vi "PostBuild.vi"(5 "Files Generated\nby Build":path[](array[path]), 6 "Top Level/Always Included VIs":path[](array[path]), 7 "Destination Path":path, 8 "error in (no error)":errorcluster, 9 "Target Name":string, 10 "Build Specification\nName":string, 11 "Project Path":path) -> (0 "error out":errorcluster)   [LabVIEW 2018]
uses:
  References/SFTP Library/Connection Info..cluster.ctl
  References/SFTP Library/Private Public Key..cluster.ctl
  References/SFTP Library/connect_key.vi
  References/SFTP Library/LabSFTP.lvlib
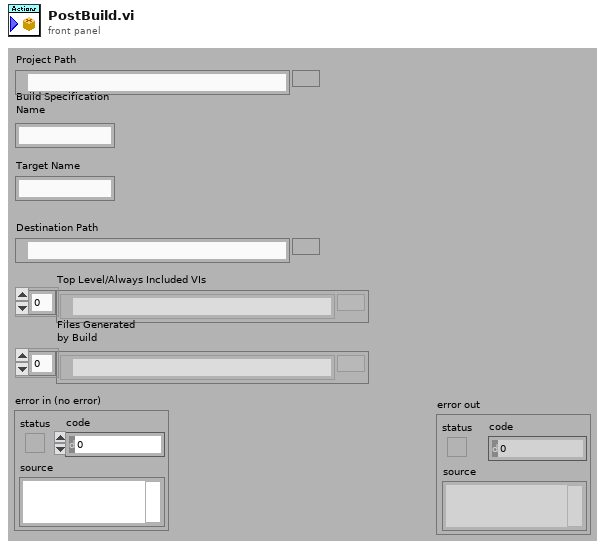
[diagram p1: front panel]
types:
  T1 = typedef "LabSFTP.lvlib/Private Public Key..cluster.ctl" = cluster{"Private Key":path, "Passphrase":string}
  T2 = typedef "LabSFTP.lvlib/Connection Info..cluster.ctl" = cluster{"Remote":string, "Username":string, "Port (22)":i32}
  T3 = enum16{"open", "replace", "create", "open or create", "replace or create", "replace or create with confirmation"}
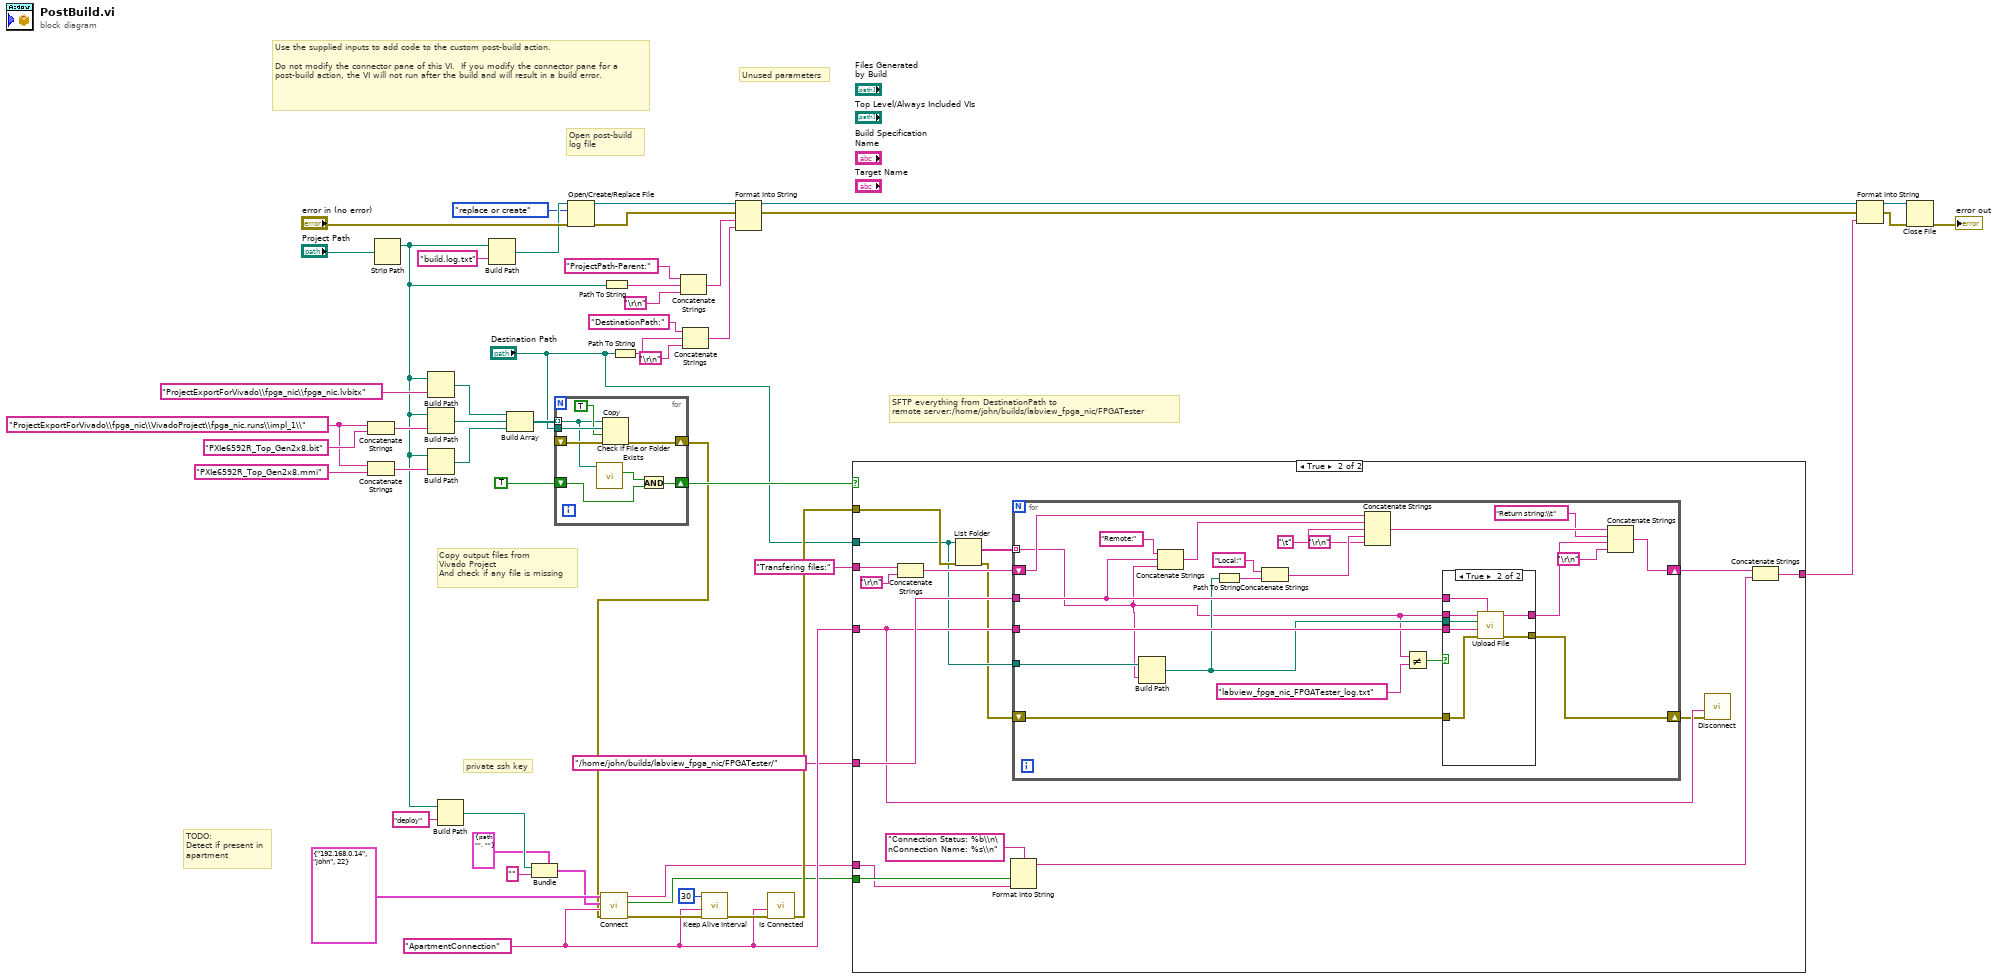
[diagram p0: block diagram]
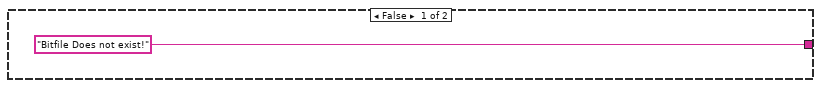
[diagram p2: hidden frame]
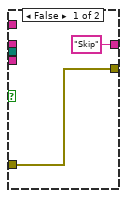
[diagram p3: hidden frame]
diagram:
  w16 = "ProjectExportForVivado\\fpga_nic\\VivadoProject\\fpga_nic.runs\\impl_1\\"
  w26 = "ApartmentConnection" ("Connection Name")
  # "private ssh key"
  # "SFTP everything from DestinationPath to\nremote server:/home/john/builds/labview_fpga_nic/FPGATester"
  # "TODO:\nDetect if present in\napartment"
  # "Unused parameters"
  # "Open post-build\nlog file"
  # "Copy output files from \nVivado Project\nAnd check if any file is missing"
  # "Use the supplied inputs to add code to the custom post-build action.\n\nDo not modify the connector pane of this VI.  If you modify the connector pane for a post-build action, the VI will not run after the build and will result in a build error."
  n1 = Concatenate Strings(w16, "PXIe6592R_Top_Gen2x8.bit") -> (w14:string)
  n2 = Concatenate Strings(w16, "PXIe6592R_Top_Gen2x8.mmi") -> (w13:string)
  n3 = Strip Path(path="Project Path") -> (stripped path=w4:path)  [unwired: 1 out]
  n4 = Build Path(base path=w4, name or relative path="ProjectExportForVivado\\fpga_nic\\fpga_nic.lvbitx") -> (appended path=w6:path)
  n5 = Build Path(base path=w4, name or relative path=w14) -> (appended path=w12:path)
  n6 = Build Path(base path=w4, name or relative path=w13) -> (appended path=w11:path)
  n7 = Build Path(base path=w4, name or relative path="deploy") -> (appended path=w21:path)
  n8 = Build Path(base path=w4, name or relative path="build.log.txt") -> (appended path=w37:path)
  n9 = Build Array(w6, w12, w11) -> (w10:path[])
  n10 = Bundle(cluster=T1 {"Private Key"=path "", "Passphrase"=""} ("Private_Public Key"), "Private Key"=w21, "Passphrase"="") -> (w19:T1)
  n11 = for {
    tunnel: w10 -> [w55] mode=indexing
    tunnel: "Destination Path" -> [w59]
    shift-right: [w57] -> w2
    shift-left: _ -> [w56]
    shift-right: [w54] -> w5
    shift-left: TRUE -> [w53]
    n12 = call <vilib>:"Check if File or Folder Exists.vi"("path"=w55) -> ("file or folder exists?"=w52:bool)  [unwired: 8 in, 2 out]
    n13 = Copy(8:w56, 9:TRUE ("overwrite (F)"), 10:w59, 11:w55) -> (0:w57:errorcluster)  [unwired: 1 in, 2 out]
    n14 = And(x=w52, y=w53) -> (x .and. y?=w54:bool)
  }
  n15 = Open/Create/Replace File(file path (use dialog)=w37, error in="error in (no error)", operation (0:open)=T3."replace or create") -> (refnum out=w50:refnum<file>, error out=w51:errorcluster)  [unwired: 3 in, 1 out]
  n16 = call-poly "Connect.vi"("error in (no error)"=w2, "Connection Name"=w26, "Private_Public Key"=w19, "Connection Info."=T2 {"Remote"="192.168.0.14", "Username"="john", "Port (22)"=22}) -> ("error out"=w30:errorcluster, "isSshConnected"=w23:bool, "Return String"=w24:string)  [unwired: 5 in]
  n17 = Path To String(path=w4) -> (string=w47:string)
  n18 = Path To String(path="Destination Path") -> (string=w43:string)
  n19 = Concatenate Strings("ProjectPath-Parent:", w47, "\r\n") -> (w3:string)
  n20 = Concatenate Strings("DestinationPath:", w43, "\r\n") -> (w8:string)
  n21 = call "Keep Alive Interval.vi"("error in (no error)"=w30, "Connection Name"=w26, "Keep Alive Interval (s)"=30) -> ("error out"=w28:errorcluster)  [unwired: 8 in]
  n22 = Format Into String(initial string=w50, error in=w51, w3, w8) -> (resulting string=w49:refnum<file>, error out=w45:errorcluster)  [unwired: 1 in]
  n23 = call "Is Connected.vi"("error in (no error)"=w28, "Connection Name"=w26) -> ("error out"=w27:errorcluster)  [unwired: 8 in, 1 out]
  n24 = case shown="True" w5 {
    tunnel: "Destination Path" -> [_ w66]
    tunnel: "Transfering files:" -> [_ w74]
    tunnel: ["Bitfile Does not exist!" w67] -> w9
    tunnel: w27 -> [_ w71]
    tunnel: w26 -> [_ w69]
    tunnel: "/home/john/builds/labview_fpga_nic/FPGATester/" -> [_ w70]
    tunnel: w23 -> [_ w68]
    tunnel: w24 -> [_ w64]
    frame False {
    }
    frame True {
      n25 = Concatenate Strings(w74, "\r\n") -> (w72:string)
      n26 = List Folder(path=w66, error in=w71) -> (filenames=w76:string[], error out=w62:errorcluster)  [unwired: 2 in, 2 out]
      n27 = Format Into String(format string="Connection Status: %b\\n\nConnection Name: %s\\n", w68, w64) -> (resulting string=w63:string)  [unwired: 2 in, 1 out]
      n28 = for {
        tunnel: w76 -> [w79] mode=indexing
        shift-right: [w85] -> w75
        shift-left: w72 -> [w98]
        tunnel: w69 -> [w97]
        tunnel: w70 -> [w94]
        tunnel: w66 -> [w96]
        shift-right: [w80] -> w61
        shift-left: w62 -> [w82]
        n29 = Build Path(base path=w96, name or relative path=w79) -> (appended path=w93:path)
        n30 = Concatenate Strings("Remote:" ("string"), w94, w79) -> (w90:string)
        n31 = Path To String(path=w93) -> (string=w92:string)
        n32 = Concatenate Strings("Local:" ("string"), w92) -> (w89:string)
        n33 = Concatenate Strings(w98, w90, "\t", w89, "\r\n") -> (w86:string)
        n34 = Not Equal?(x=w79, y="labview_fpga_nic_FPGATester_log.txt") -> (x != y?=w78:bool)
        n35 = case shown="True" w78 {
          tunnel: w97 -> [_ w107]
          tunnel: w94 -> [_ w106]
          tunnel: w79 -> [_ w105]
          tunnel: w93 -> [_ w104]
          tunnel: w82 -> [w99 w103]
          tunnel: ["Skip" ("Return String") w102] -> w81
          tunnel: [w99 w101] -> w80
          frame False {
          }
          frame True {
            n36 = call "Upload File.vi"("Remote Folder Path"=w106, "error in (no error)"=w103, "Connection Name"=w107, "Local File Path"=w104, "Remote File Name"=w105) -> ("error out"=w101:errorcluster, "Return String"=w102:string)  [unwired: 5 in]
          }
        }
        n37 = Concatenate Strings(w86, "Return string:\\t" ("string"), w81, "\r\n") -> (w85:string)
      }
      n38 = call "Disconnect.vi"("error in (no error)"=w61, "Connection Name"=w69) -> ()  [unwired: 7 in, 3 out]
      n39 = Concatenate Strings(w75, w63) -> (w67:string)
    }
  }
  n40 = Format Into String(initial string=w49, error in=w45, w9) -> (resulting string=w34:refnum<file>, error out=w33:errorcluster)  [unwired: 1 in]
  n41 = Close File(refnum=w34, error in=w33) -> (error out=→"error out":errorcluster)  [unwired: 1 out]
